vi "Data of the Joystick.vi"(8 "error in (no error)":errorcluster, 11 "device ID":refnum<k1>) -> (0 "error out":errorcluster, 2 "Joystick":T1={"L Stick"=FALSE, "R Stick"=FALSE, "X"=FALSE, "A"=FALSE, "Y"=FALSE, "B"=FALSE, "45"=FALSE, "90"=FALSE, "135"=FALSE, "180"=FALSE, "225"=FALSE, "270"=FALSE, "315"=FALSE, "0"=FALSE, "Start"=FALSE, "Back"=FALSE, "RB"=FALSE, "LB"=FALSE, "X Right"=0, "Y Right"=0, "X Left"=0, "Y Left"=0, "Z Right"=0, "Pov"=-1, "Z Left"=0, "Num"=0} {"Z Right" scale=0.0..100.0; "Y Left" scale=-100.0..100.0; "X Left" scale=-100.0..100.0; "Y Right" scale=-100.0..100.0; "X Right" scale=-100.0..100.0}, 3 "device ID out":refnum<k1>)   [LabVIEW 2020]
uses:
  Joystick controls.ctl
  <vilib>/Utility/inputDevices.llb/joystickAcquire.vi
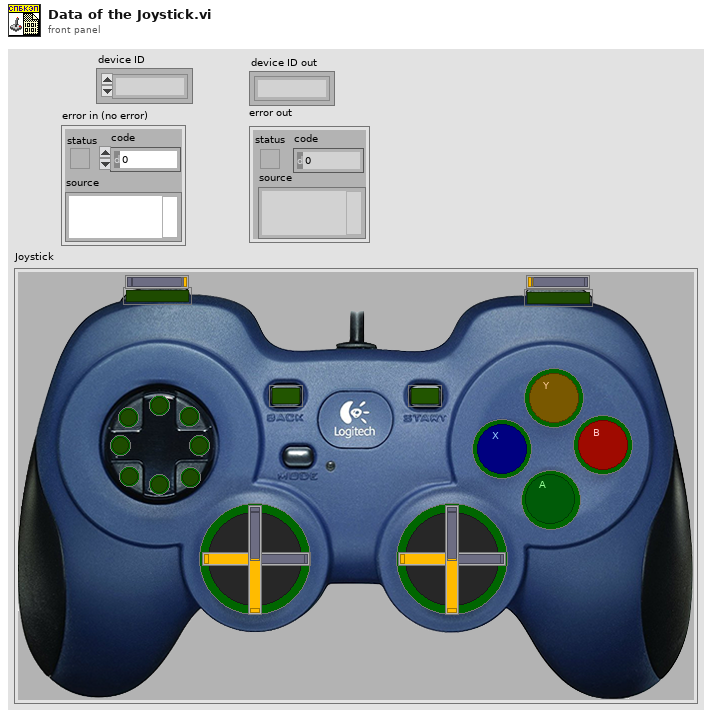
[diagram p1: front panel]
types:
  T1 = typedef "Joystick controls.ctl" = cluster{"L Stick":bool, "R Stick":bool, "X":bool, "A":bool, "Y":bool, "B":bool, "45":bool, "90":bool, "135":bool, "180":bool, "225":bool, "270":bool, "315":bool, "0":bool, "Start":bool, "Back":bool, "RB":bool, "LB":bool, "X Right":i8, "Y Right":i8, "X Left":i8, "Y Left":i8, "Z Right":i8, "Pov":i16, "Z Left":i8, "Num":i16}
  T2 = cluster{"X axis":i32, "Y axis":i32, "Z axis":i32, "X axis rotation":i32, "Y axis rotation":i32, "Z axis rotation":i32, "U axis":i32, "V axis":i32}
  T3 = cluster{"button 1":bool, "button 2":bool, "button 3":bool, "button 4":bool, "button 5":bool, "button 6":bool, "button 7":bool, "button 8":bool, "button 9":bool, "button 10":bool, "button 11":bool, "button 12":bool, "button 13":bool, "button 14":bool, "button 15":bool, "button 16":bool, "button 17":bool, "button 18":bool, "button 19":bool, "button 20":bool, "button 21":bool, "button 22":bool, "button 23":bool, "button 24":bool, "button 25":bool, "button 26":bool, "button 27":bool, "button 28":bool, "button 29":bool, "button 30":bool, "button 31":bool, "button 32":bool}
  T4 = cluster{"pov 1":i32, "pov 2":i32, "pov 3":i32, "pov 4":i32}
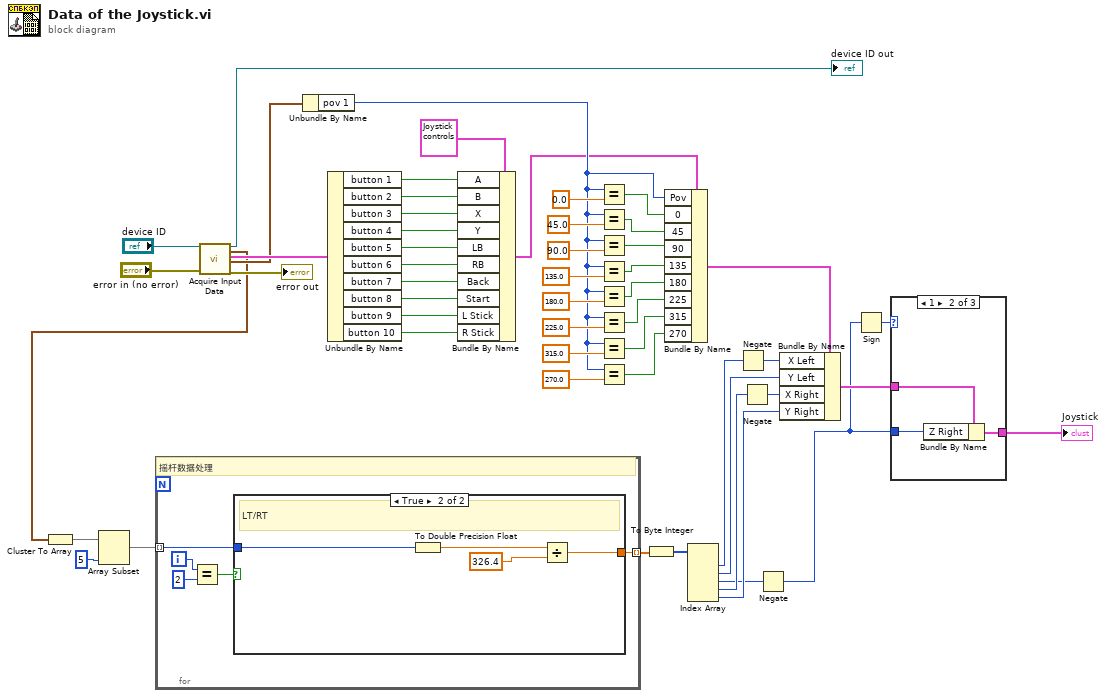
[diagram p0: block diagram]
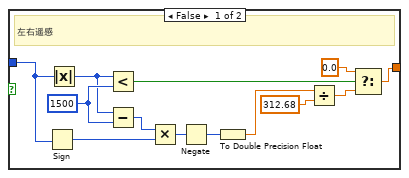
[diagram p2: hidden frame]
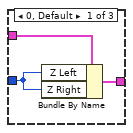
[diagram p3: hidden frame]
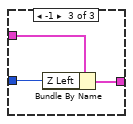
[diagram p4: hidden frame]
diagram:
  n1 = call-poly <vilib>:"Acquire Input Data.vi"("device ID"="device ID", "error in (no error)"="error in (no error)") -> ("device ID"=→"device ID out":refnum<k1>, "axis info"=w13:T2, "button info"=w51:T3, "direction info"=w40:T4, "error out"=→"error out":errorcluster)  [unwired: 13 in]
  n2 = Cluster To Array(cluster=w13) -> (array=w16:i32[])
  n3 = Array Subset(array=w16, length=5 ("长度")) -> (w14:i32[])  [unwired: 1 in]
  n4 = for {
    tunnel: w14 -> [w58] mode=indexing
    tunnel: [w54] -> w4 mode=indexing
    i -> [w57]
    # "摇杆数据处理"
    n5 = Equal?(x=w57, y=2) -> (x = y?=w55:bool)
    n6 = case shown="True" w55 {
      tunnel: w58 -> [w61 w74]
      tunnel: [w69 w72] -> w54
      frame False {
        w68 = 1500 ("y")
        # "左右遥感"
        n7 = Sign(1:w61) -> (0:w66:i32)
        n8 = Absolute Value(x=w61) -> (abs(x)=w63:i32)
        n9 = Less?(x=w63, y=w68) -> (x < y?=w71:bool)
        n10 = Subtract(x=w63, y=w68) -> (x-y=w67:i32)
        n11 = Multiply(x=w67, y=w66) -> (x*y=w65:i32)
        n12 = Negate(x=w65) -> (-x=w62:i32)
        n13 = To Double Precision Float(number=w62) -> (double precision float=w60:dbl)
        n14 = Divide(x=w60, y=312.68 ("x")) -> (x/y=w59:dbl)
        n15 = Select(t=0.0, s=w71, f=w59) -> (s? t:f=w69:dbl)
      }
      frame True {
        # "LT/RT"
        n16 = To Double Precision Float(number=w74) -> (double precision float=w73:dbl)
        n17 = Divide(x=w73, y=326.4) -> (x/y=w72:dbl)
      }
    }
  }
  n18 = Unbundle By Name(w40) -> ("pov 1"=w23:i32)
  n19 = Unbundle By Name(w51) -> ("button 1"=w50:bool, "button 2"=w49:bool, "button 3"=w48:bool, "button 4"=w47:bool, "button 5"=w46:bool, "button 6"=w45:bool, "button 7"=w44:bool, "button 8"=w43:bool, "button 9"=w42:bool, "button 10"=w41:bool)
  n20 = Bundle By Name(cluster=T1 {"L Stick"=FALSE, "R Stick"=FALSE, "X"=FALSE, "A"=FALSE, "Y"=FALSE, "B"=FALSE, "45"=FALSE, "90"=FALSE, "135"=FALSE, "180"=FALSE, "225"=FALSE, "270"=FALSE, "315"=FALSE, "0"=FALSE, "Start"=FALSE, "Back"=FALSE, "RB"=FALSE, "LB"=FALSE, "X Right"=0, "Y Right"=0, "X Left"=0, "Y Left"=0, "Z Right"=0, "Pov"=-1, "Z Left"=0, "Num"=0} ("Joystick"), "A"=w50, "B"=w49, "X"=w48, "Y"=w47, "LB"=w46, "RB"=w45, "Back"=w44, "Start"=w43, "L Stick"=w42, "R Stick"=w41) -> (w12:T1)
  n21 = Equal?(x=w23, y=0.0) -> (x = y?=w28:bool)
  n22 = Equal?(x=w23, y=45.0) -> (x = y?=w29:bool)
  n23 = Equal?(x=w23, y=90.0) -> (x = y?=w30:bool)
  n24 = Equal?(x=w23, y=135.0) -> (x = y?=w31:bool)
  n25 = Equal?(x=w23, y=180.0) -> (x = y?=w27:bool)
  n26 = Equal?(x=w23, y=225.0) -> (x = y?=w26:bool)
  n27 = Equal?(x=w23, y=315.0) -> (x = y?=w25:bool)
  n28 = Equal?(x=w23, y=270.0) -> (x = y?=w24:bool)
  n29 = To Byte Integer(number=w4) -> (8bit integer=w3:i8[])
  n30 = Bundle By Name(cluster=w12, "Pov"=w23, "0"=w28, "45"=w29, "90"=w30, "135"=w31, "180"=w27, "225"=w26, "315"=w25, "270"=w24) -> (w11:T1)
  n31 = Index Array(array=w3) -> (element #1=w8:i8, element #2=w20:i8, element #3=w6:i8, element #4=w10:i8, element #5=w19:i8)  [unwired: 5 in]
  n32 = Negate(x=w8) -> (-x=w7:i8)
  n33 = Negate(x=w10) -> (-x=w9:i8)
  n34 = Negate(x=w6) -> (-x=w5:i8)
  n35 = Bundle By Name(cluster=w11, "X Left"=w7, "Y Left"=w20, "X Right"=w9, "Y Right"=w19) -> (w17:T1)
  n36 = Sign(1:w5) -> (0:w18:i8)
  n37 = case shown="1" w18 {
    tunnel: w5 -> [w77 w81 w84]
    tunnel: w17 -> [w78 w80 w83]
    tunnel: [w76 w79 w82] -> w1
    frame 0, Default {
      n38 = Bundle By Name(cluster=w78, "Z Left"=w77, "Z Right"=w77) -> (w76:T1)
    }
    frame 1 {
      n39 = Bundle By Name(cluster=w80, "Z Right"=w81) -> (w79:T1)
    }
    frame -1 {
      n40 = Bundle By Name(cluster=w83, "Z Left"=w84) -> (w82:T1)
    }
  }
  "Joystick" <- w1
